vi "Test_IncrementValuePublication_I32_ValueIncremented.vi"(8 "error in (no error)":errorcluster, 11 "TestCase in":refnum<class "TestPublicationPolicy.lvclass">) -> (0 "error out":errorcluster, 3 "TestCase out":refnum<class "TestPublicationPolicy.lvclass">)   [LabVIEW 2020, in "TestPublicationPolicy.lvclass"]
uses:
  TestPublicationPolicy.lvclass
  TestPublicationPolicy.lvclass/TestPublicationPolicy.ctl
  Source/PublicationPolicy/IncrementValuePublication/IncrementValuePublication.lvclass
  Source/IMediator/MutexedPublishRequest/MutexedPublishRequest.lvclass
  Source/IMediator/IPublicationPolicy/IPublicationPolicy.lvclass
  modules/composed-transport/Source/Concrete/NotifierTransport/NotifierTransport.lvclass
  C:/Git/mva-core/Source/IMediator/IPublicationPolicy/IPublicationPolicy.lvclass
  C:/Git/mva-core/Source/PublicationPolicy/IncrementValuePublication/IncrementValuePublication.lvclass
  C:/Git/mva-core/modules/composed-transport/Source/ITransport/ITransport.lvclass
  C:/Git/mva-core/modules/composed-transport/Source/Concrete/NotifierTransport/NotifierTransport.lvclass
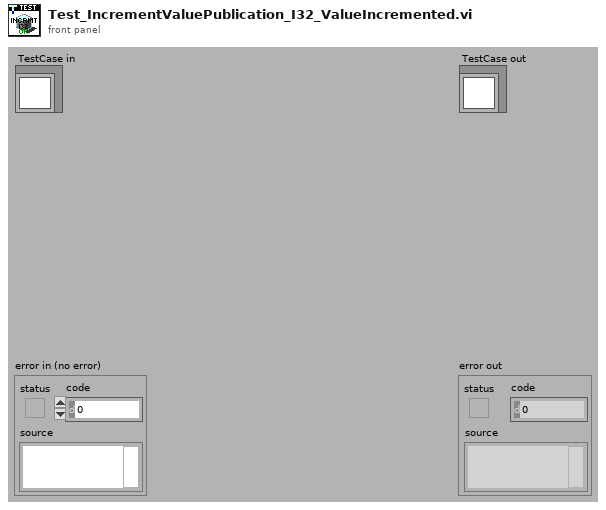
[diagram p1: front panel]
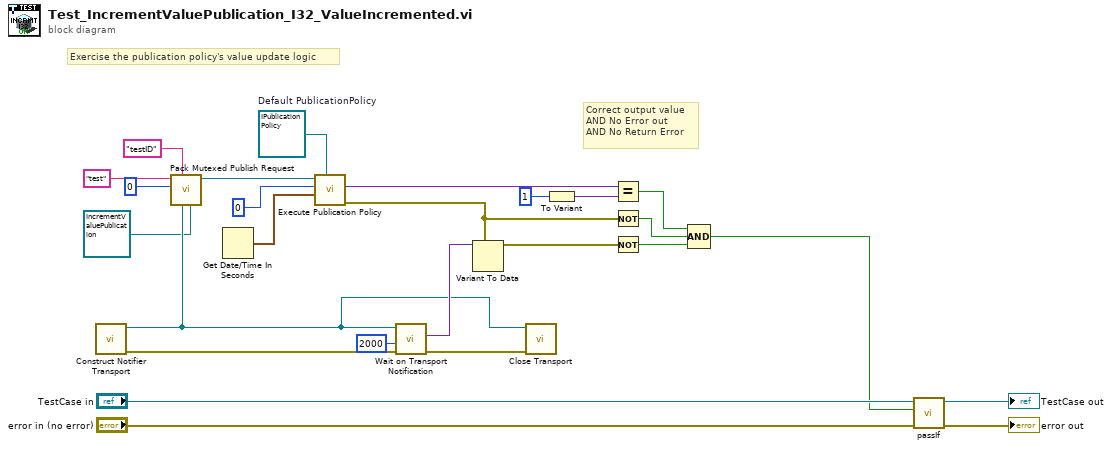
[diagram p0: block diagram]
diagram:
  w19 = refnum<class "IPublicationPolicy.lvclass"> refnum  # Default PublicationPolicy
  # "Correct output value\nAND No Error out\nAND No Return Error"
  # "Exercise the publication policy's value update logic"
  n1 = call "Construct Notifier Transport.vi"() -> ("error out"=w15:errorcluster, "NotifierTransport"=w3:refnum<class "NotifierTransport.lvclass">)  [unwired: 10 in]
  n2 = call "Pack Mutexed Publish Request.vi"("PublicationPolicy"=refnum<class "IncrementValuePublication.lvclass"> refnum ("PublicationPolicy.lvlib:IncrementValuePublication.lvclass"), "Return Error Transport"=w3, "Publisher ID"="testID", "Datum Value or Type"=0 ("Data to Publish"), "Datum Name"="test") -> ("MutexedPublishRequest Out"=w20:refnum<class "MutexedPublishRequest.lvclass">)  [unwired: 5 in, 1 out]
  n3 = Get Date/Time In Seconds() -> (seconds since 1Jan1904=w21:timestamp)
  n4 = call-dynamic "Execute Publication Policy.vi"("Default PublicationPolicy"=w19, "Last Publish Time"=w21, "Last Published Value"=0, "MutexedPublishRequest"=w20) -> ("error out (Reject Publication)"=w5:errorcluster, "Value to Publish"=w12:variant)  [unwired: 5 in, 1 out]
  n5 = call "Wait on Transport Notification.vi"("error in (no error)"=w15, "Timeout In ms (-1)"=2000, "NotifierTransport"=w3) -> ("error out"=w2:errorcluster, "Data"=w13:variant)  [unwired: 6 in, 1 out]
  n6 = Variant To Data(type=w5, Variant=w13) -> (data=w9:errorcluster)  [unwired: 1 in, 1 out]
  n7 = call-dynamic "Close Transport.vi"("error in (no error)"=w2, "NotifierTransport"=w3) -> ()  [unwired: 9 in, 1 out]
  n8 = To Variant(anything=1) -> (Variant=w10:variant)
  n9 = Equal?(x=w12, y=w10) -> (x = y?=w8:bool)
  n10 = Not(x=w5) -> (.not. x?=w4:bool)
  n11 = Not(x=w9) -> (.not. x?=w6:bool)
  n12 = Compound Arithmetic op=AND(w8, w4, w6) -> (w7:bool)
  n13 = call-dynamic "passIf.vi"("error in (no error)"="error in (no error)", "pass"=w7, "TestCase in"="TestCase in") -> ("error out"=→"error out":errorcluster, "TestCase out"=→"TestCase out":refnum<class "TestPublicationPolicy.lvclass">)  [unwired: 7 in]
